vi "op_biti_v3.vi"() -> ()   [LabVIEW 2010]
panel:
  out "Val_shift":dbl=154.0
  in  "Nr biti":i8=1
  out "Array 2":bool[](array[boolean])=[TRUE, FALSE, FALSE, TRUE, TRUE, FALSE, TRUE, FALSE]
  in  "Val num":u8=77
  out "Array":bool[](array[boolean])=[FALSE, TRUE, FALSE, FALSE, TRUE, TRUE, FALSE, TRUE]
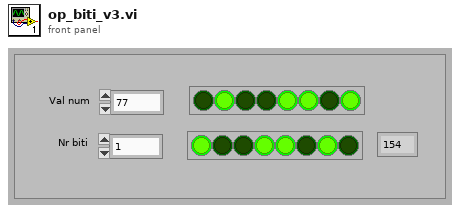
[diagram p1: front panel]
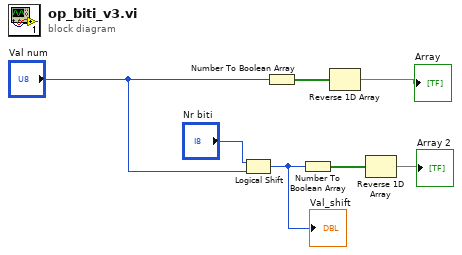
[diagram p0: block diagram]
diagram:
  n1 = Logical Shift(y="Nr biti", x="Val num") -> (x << y=w1:u8)
  "Val_shift" <- w1
  n2 = Number To Boolean Array(number="Val num") -> (Boolean array=w7:bool[])
  n3 = Number To Boolean Array(number=w1) -> (Boolean array=w5:bool[])
  n4 = Reverse 1D Array(array=w7) -> (reversed array=→"Array":bool[])
  n5 = Reverse 1D Array(array=w5) -> (reversed array=→"Array 2":bool[])
